vi "LidarSerialReadWrite.vi"(11 "SelectLIDAR":enum16{"Raphael", "Leonardo"}(ring)) -> ()   [LabVIEW 2010]
doc: "LidarSerialReadWrite.vi uses the FGPA DIO to read and write serial data with the LIDAR. Data to send to the LIDAR is read from a FIFO, and data read from the LIDAR is written to a FIFO for later processing.\n\n<b>Inputs</b>\nSelectLIDAR - selects which LIDAR to talk to"
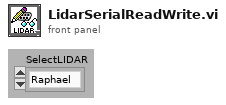
[diagram p1: front panel]
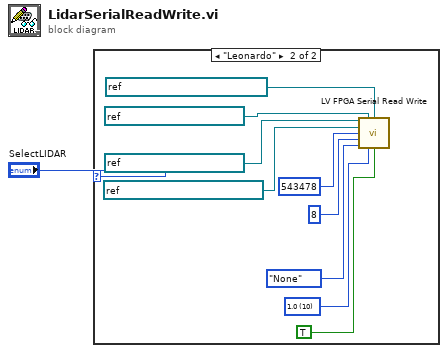
[diagram p0: block diagram]
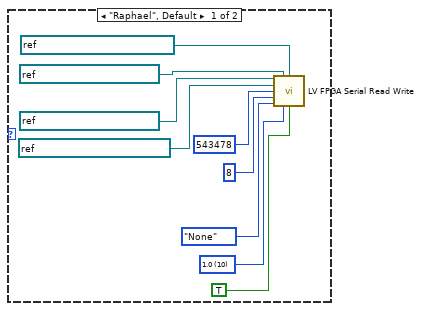
[diagram p2: hidden frame]
diagram:
  n1 = case shown="\"Leonardo\"" "SelectLIDAR" {
    frame "Raphael", Default {
      w10 = u16 10 items=["1.0"=10, "1.5"=15, "2.0"=20] ("stop bits (10: 1 bit)")
      n2 = call "LV FPGA Serial Read Write.vi"("Transmit"=refnum<k21> "Chassis1/Mod1/DIO2", "Receive"=refnum<k21> "Chassis1/Mod1/DIO4", "Write FIFO"=refnum<k21> "LIDARRaphaelWriteFIFO", "Read FIFO"=refnum<k21> "LIDARRaphaelReadFIFO", "baud rate (9600)"=u32 543478, "data bits (8)"=8, "parity (0:none)"=enum16{"None", "Odd", "Even", "Mark", "Space"}."None", "stop bits (10: 1 bit)"=w10, "Invert Polarity?"=TRUE) -> ()  [unwired: 7 in]
    }
    frame "Leonardo" {
      w19 = u16 10 items=["1.0"=10, "1.5"=15, "2.0"=20] ("stop bits (10: 1 bit)")
      n3 = call "LV FPGA Serial Read Write.vi"("Transmit"=refnum<k21> "Chassis1/Mod1/DIO3", "Receive"=refnum<k21> "Chassis1/Mod1/DIO5", "Write FIFO"=refnum<k21> "LIDARLeonardoWriteFIFO", "Read FIFO"=refnum<k21> "LIDARLeonardoReadFIFO", "baud rate (9600)"=u32 543478, "data bits (8)"=8, "parity (0:none)"=enum16{"None", "Odd", "Even", "Mark", "Space"}."None", "stop bits (10: 1 bit)"=w19, "Invert Polarity?"=TRUE) -> ()  [unwired: 7 in]
    }
  }
